vi "_script_enable_run_when_opened.vi"() -> (0 "error out":errorcluster)   [LabVIEW 2017]
uses:
  _Shared/CSM Shared.lvlib
panel:
  out "filenames":string[](array[string])
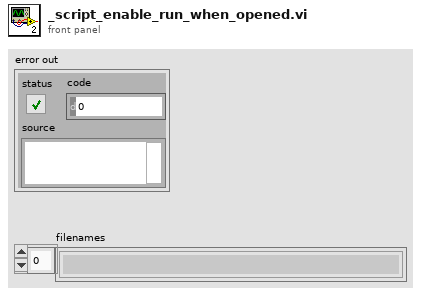
[diagram p1: front panel]
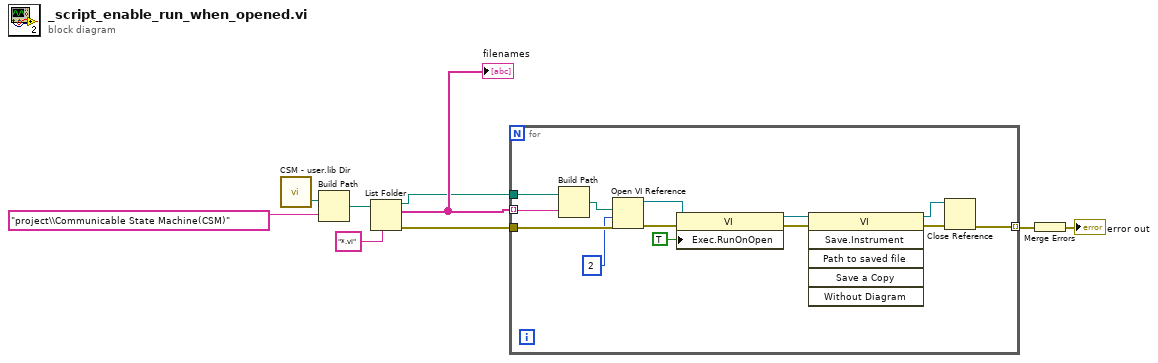
[diagram p0: block diagram]
diagram:
  n1 = call "CSM - user.lib Dir.vi"() -> ("<LabVIEW>"=w8:path)  [unwired: 2 in, 1 out]
  n2 = Build Path(base path=w8, name or relative path="project\\Communicable State Machine(CSM)") -> (appended path=w7:path)
  n3 = List Folder(path=w7, pattern="*.vi") -> (path out=w3:path, filenames=w4:string[], error out=w5:errorcluster)  [unwired: 2 in, 1 out]
  "filenames" <- w4
  n4 = for {
    tunnel: [w15] -> w2 mode=indexing
    tunnel: w5 -> [w14]
    tunnel: w4 -> [w11] mode=indexing
    tunnel: w3 -> [w12]
    n5 = Build Path(base path=w12, name or relative path=w11) -> (appended path=w13:path)
    n6 = Open VI Reference(vi path=w13, options=2, error in (no error)=w14) -> (vi reference=w22:refnum<vi>, error out=w19:errorcluster)  [unwired: 3 in]
    n7 = property class="VI"(reference=w22, error in=w19, "Exec.RunOnOpen"=TRUE ("Execution:Run When Opened")) -> (reference out=w21:refnum<vi>, error out=w20:errorcluster)
    n8 = invoke class="VI" method="Save.Instrument"(reference=w21, error in=w20) -> (reference out=w16:refnum<vi>, error out=w17:errorcluster)  [unwired: 4 in, 4 out]
    n9 = Close Reference(reference=w16, error in (no error)=w17) -> (error out=w15:errorcluster)
  }
  n10 = Merge Errors(w2) -> (→"error out":errorcluster)
